vi "Test Animal Cannot Eat after Eating.vi"(8 "error in (no error)":errorcluster, 11 "Hungry Hippo Test In":refnum<class "Hungry Hippo Test.lvclass">) -> (0 "error out":errorcluster, 3 "Hungry Hippo Test Out":refnum<class "Hungry Hippo Test.lvclass">)   [LabVIEW 2020, in "Hungry Hippo Test.lvclass"]
doc: "Override of Test Animal Cannot Eat After Eating.\nThe Hungry Hippo can always eat."
uses:
  Hungry Hippo Test.lvclass
  C:/Program Files (x86)/National Instruments/LabVIEW 2020/vi.lib/Astemes/LUnit/Test Case.lvclass
  <vilib>/Astemes/LUnit/Test Case.lvclass/Test Case.ctl
  <vilib>/Astemes/LUnit/Test Case.lvclass
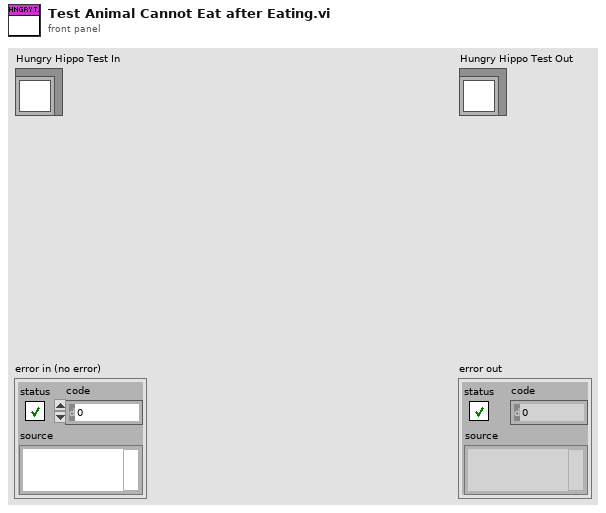
[diagram p1: front panel]
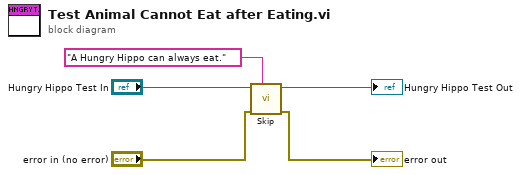
[diagram p0: block diagram]
diagram:
  n1 = call <vilib>:"Skip.vi"("Description"="A Hungry Hippo can always eat.", "error in (no error)"="error in (no error)", "LUnit Test Case In"="Hungry Hippo Test In") -> ("error out"=→"error out":errorcluster, "LUnit Test Case Out"=→"Hungry Hippo Test Out":refnum<class "Hungry Hippo Test.lvclass">)  [unwired: 7 in]
